vi "Num Events.vi"(8 "error in (no error)":errorcluster, 11 "EventMgr in":refnum<class "EventMgr.lvclass">) -> (0 "error out":errorcluster, 2 "Number Unflushed Events":i32, 3 "EventMgr out":refnum<class "EventMgr.lvclass">)   [LabVIEW 2013, in "EventMgr.lvclass"]
uses:
  EventMgr.lvclass
  EventMgr.lvclass/EventMgr.ctl
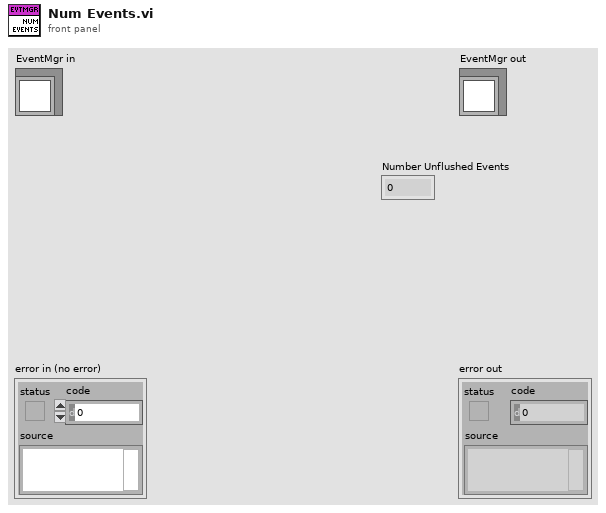
[diagram p1: front panel]
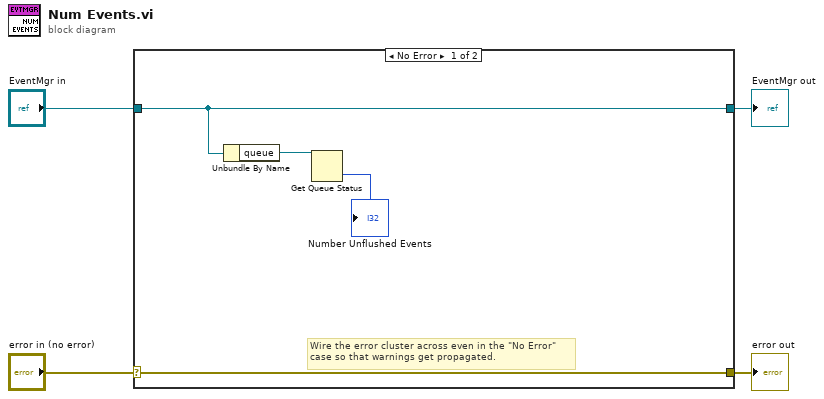
[diagram p0: block diagram]
diagram:
  n1 = case shown="No Error" "error in (no error)" {
    selector: "error in (no error)" -> [w8 w10]
    tunnel: [w8 w10] -> w3
    tunnel: [w7 w9] -> w1
    tunnel: "EventMgr in" -> [w7 w9]
    frame No Error {
      # "Wire the error cluster across even in the \"No Error\"\ncase so that warnings get propagated."
      n2 = Unbundle By Name(w7) -> ("queue"=w6:refnum<queue>)
      n3 = Get Queue Status(queue=w6) -> (# elements in queue=→"Number Unflushed Events":i32)  [unwired: 2 in, 7 out]
    }
    frame Error {
    }
  }
  "error out" <- w3
  "EventMgr out" <- w1
